vi "VariavelGlobalTDD.vi"() -> ()   [LabVIEW 2012]
panel:
  in  "Boolean 2":bool
  out "Boolean":bool
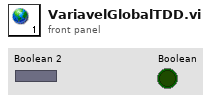
[diagram p1: front panel]
diagram:
